vi "savetxt.vi"(9 "2D data":dbl[][](array[numeric])=[[0.0, 1.0], [2.0, 3.0]] caption="matrix" format="%0.2f", 10 "name":string="temperary", 11 "path":path=path "I:/Test") -> (0 "saved path":path=path "I:/Test/temperary.txt")   [LabVIEW 2020]
uses:
  <vilib>/Utility/file.llb/Write Delimited Spreadsheet (DBL).vi
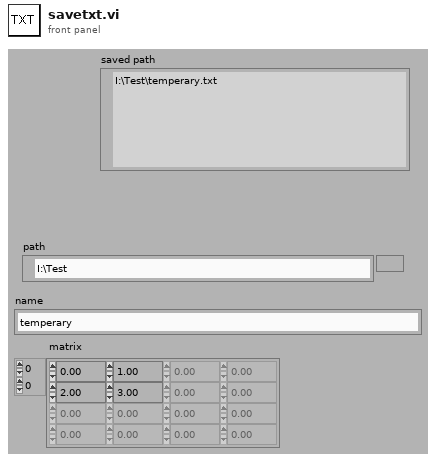
[diagram p1: front panel]
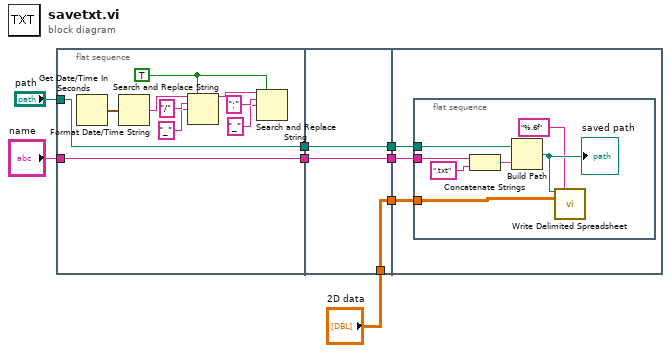
[diagram p0: block diagram]
diagram:
  n1 = flat-sequence {
    tunnel: [w9] -> w8
    tunnel: [w11] -> w7
    tunnel: "path" -> [w11]
    tunnel: "name" -> [w9]
    tunnel: w8 -> [w21]
    tunnel: [w21] -> w6
    tunnel: w7 -> [w20]
    tunnel: [w20] -> w5
    tunnel: [w19] -> w4
    tunnel: "2D data" -> [w19]
    tunnel: w6 -> [w24]
    tunnel: w5 -> [w23]
    tunnel: w4 -> [w22]
    frame #0 {
      w10 = TRUE ("replace all? (F)")
      n2 = Get Date/Time In Seconds() -> (seconds since 1Jan1904=w12:timestamp)
      n3 = Format Date/Time String(seconds (now)=w12) -> (date/time string=w18:string)  [unwired: 2 in]
      n4 = Search and Replace String(replace all?=w10, input string=w18, search string="/" ("搜索字符串"), replace string="_" ("替换字符串(\"\")")) -> (result string=w15:string)  [unwired: 1 in, 6 out]
      n5 = Search and Replace String(replace all?=w10, input string=w15, search string=":" ("搜索字符串"), replace string="_" ("替换字符串(\"\")")) -> ()  [unwired: 1 in, 7 out]
    }
    frame #1 {
    }
    frame #2 {
      n6 = flat-sequence {
        tunnel: w24 -> [w31]
        tunnel: w23 -> [w28]
        tunnel: w22 -> [w26]
        frame #0 {
          n7 = Concatenate Strings(w31, ".txt" ("搜索字符串")) -> (w29:string)
          n8 = Build Path(base path=w28, name or relative path=w29) -> (appended path=w27:path)
          "saved path" <- w27
          n9 = call-poly <vilib>:"Write Delimited Spreadsheet.vi"("file path (dialog if empty)"=w27, "format (%.3f)"="%.6f", "2D data"=w26) -> ()  [unwired: 11 in, 2 out]
        }
      }
    }
  }
